vi "Init.vi"(11 "Mine in":refnum<class "Mine.lvclass">) -> (3 "Mine out":refnum<class "Mine.lvclass">)   [LabVIEW 2023, in "d19.lvlib" / "Mine.lvclass"]
uses:
  Mine.lvclass
  Mine.lvclass/Mine.ctl
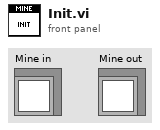
[diagram p1: front panel]
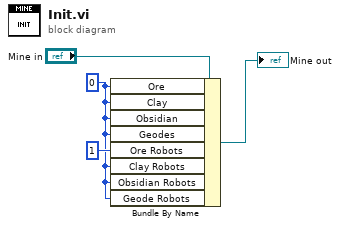
[diagram p0: block diagram]
diagram:
  w1 = u8 0 ("Clay Robots")
  n1 = Bundle By Name(cluster="Mine in", "Ore"=w1, "Clay"=w1, "Obsidian"=w1, "Geodes"=w1, "Ore Robots"=u8 1, "Clay Robots"=w1, "Obsidian Robots"=w1, "Geode Robots"=w1) -> (→"Mine out":refnum<class "Mine.lvclass">)
